vi "FTW-JSON-Core-GetFlattenedValue.vi"(0 "JSON Library Filepath":path, 5 "JSON Element":i64 format="%016x", 7 "LabVIEW Type":T1, 9 "Element Default Value":variant, 11 "error in":errorcluster, 12 "Encoding Flags":i64 format="%016x") -> (4 "Flattened Value":string, 15 "error out":errorcluster)   [LabVIEW 2014]
uses:
  reflection/FTW-Reflection-Types.ctl
  FTW-JSON-Core-Type.ctl
  error/FTW-ERR-ThrowError.vi
  lib/jansson/FTWLib-JSON-LibraryFilepath.vi
  error/FTW-ERR-NoErrorConstant.vi
  error/FTW-ERR-CallChain.vi
  string/FTW-STR-ReplaceWhitespace.vi
panel:
  # "Inputs"
  # "Outputs"
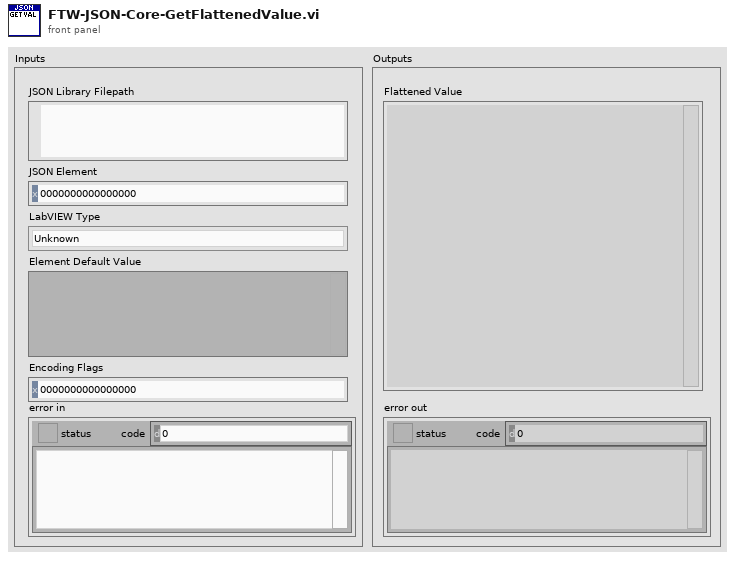
[diagram p1: front panel]
types:
  T1 = typedef "FTW-Reflection-Types.ctl" = enum16{"Unknown", "Void", "Array", "Cluster", "LVObject", "Boolean", "I8", "I16", "I32", "I64", "U8", "U16", "U32", "U64", "SGL", "DBL", "EXT", "CSG", "CDB", "CXT", "FXP", "EnumU8", "EnumU16", "EnumU32", "EnumU64", "SGLwithUnit", "DBLwithUnit", "EXTwithUnit", "CSGwithUnit", "CDBwithUnit", "CXTwithUnit", "String", "Path", "Picture", "Tag", "LVVariant", "Timestamp", "WaveformI8", "WaveformI16", "WaveformI32", "WaveformI64", "WaveformU8", "WaveformU16", "WaveformU32", "WaveformU64", "WaveformSGL", "WaveformDBL", "WaveformEXT", "WaveformCSG", "WaveformCDB", "WaveformCXT", "WaveformDigital", "WaveformUnknownType", "DigitalData", "DynamicData", "ExternalData", "FileByteStream", "TDMStream", "dotNET", "ActiveX", "VIServerReference", "VIReference", "ApplicationInstance", "Menu", "ConnectionDataSocket", "ConnectionVISA", "ConnectionBluetooth", "ConnectionIrDA", "ConnectionTCP", "ConnectionUDP", "ConnectionHTTPClient", "ConnectionFTP", "Occurrence", "Notifier", "Queue", "Rendezvous", "Semaphore", "RTFIFO", "EventPublisher", "EventRegistration", "EventCallback", "DataValueReference", "GenericClass", "GenericClassTag", "GenericClassDeepCopy", "GenericClassFlattened", "GenericClassTagFlattened", "GenericReferenceType", "WindowsRegistry", "OverloadedDatalogRef", "ReferenceUnknownType"}
  T2 = typedef "FTW-JSON-Core-Type.ctl" = enum16{"Object", "Array", "String", "Integer", "Floating Point", "true", "false", "null", "undefined"}
  T3 = cluster{"Element Name":string, "Element Type":T1, "Element Value":variant}[]
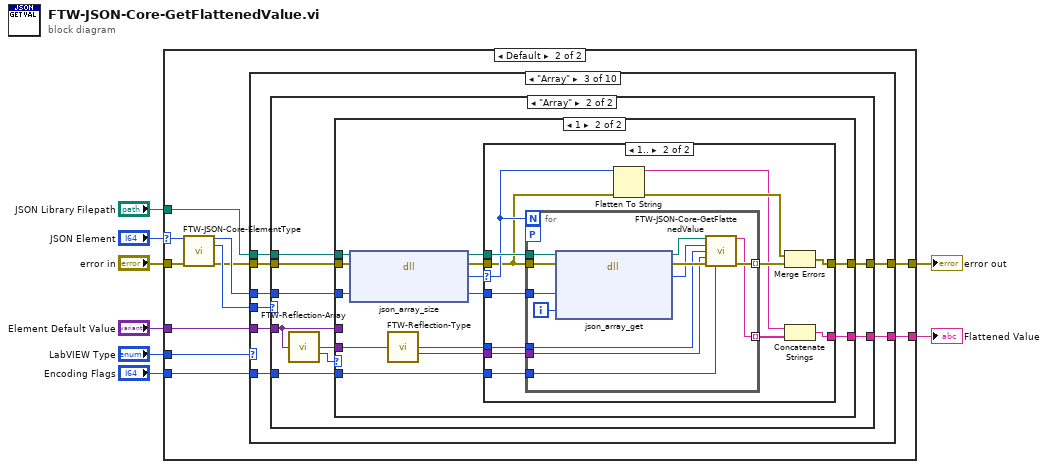
[diagram p0: block diagram]
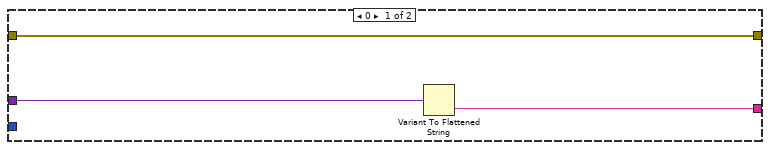
[diagram p2: hidden frame]
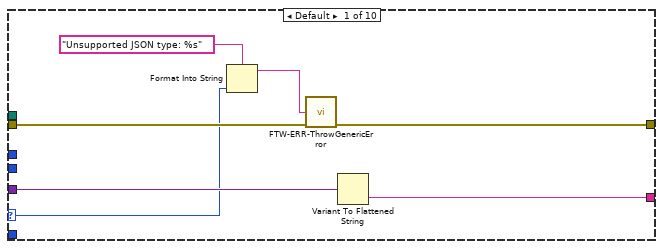
[diagram p3: hidden frame]
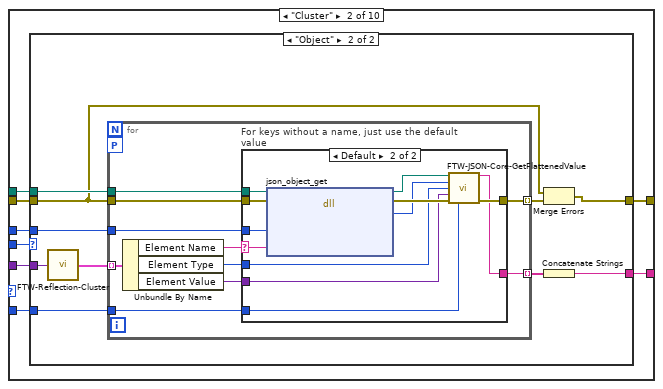
[diagram p4: hidden frame]
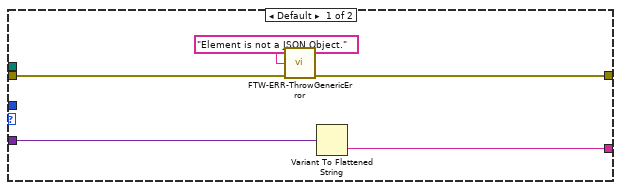
[diagram p5: hidden frame]
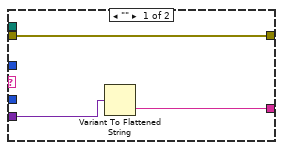
[diagram p6: hidden frame]
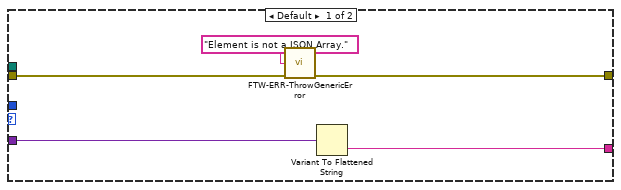
[diagram p7: hidden frame]
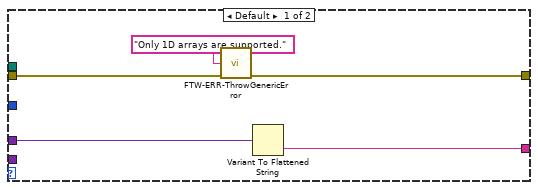
[diagram p8: hidden frame]
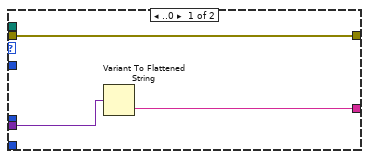
[diagram p9: hidden frame]
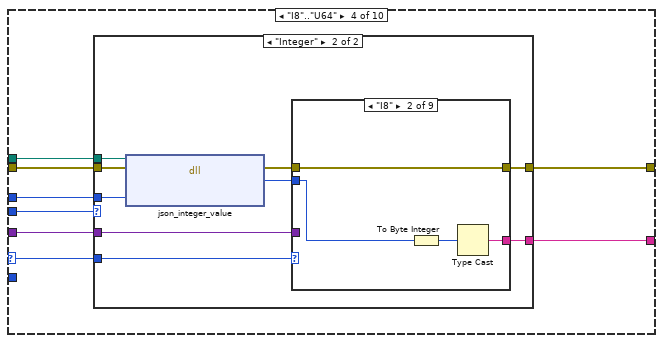
[diagram p10: hidden frame]
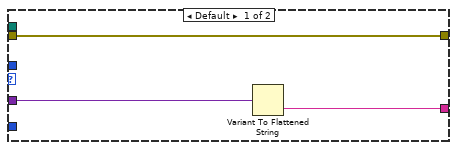
[diagram p11: hidden frame]
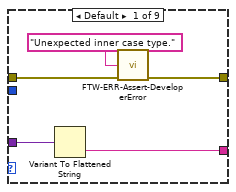
[diagram p12: hidden frame]
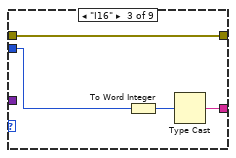
[diagram p13: hidden frame]
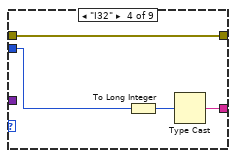
[diagram p14: hidden frame]
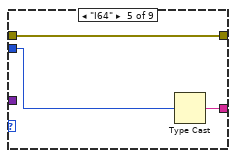
[diagram p15: hidden frame]
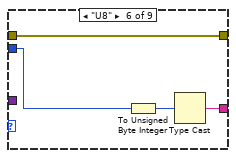
[diagram p16: hidden frame]
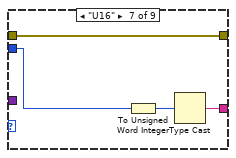
[diagram p17: hidden frame]
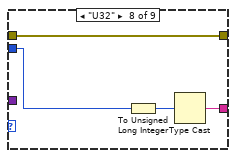
[diagram p18: hidden frame]
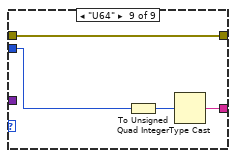
[diagram p19: hidden frame]
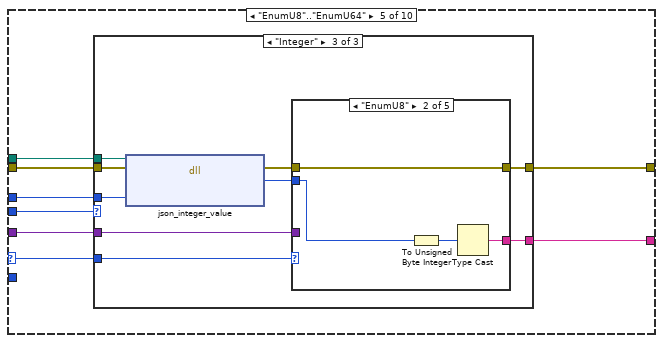
[diagram p20: hidden frame]
diagram:
  n1 = case shown="Default" "JSON Element" {
    selector: "JSON Element" -> [_ w15]
    tunnel: [w9 w22] -> w8
    tunnel: [w10 w21] -> w6
    tunnel: "LabVIEW Type" -> [_ w20]
    tunnel: "Element Default Value" -> [w11 w19]
    tunnel: "error in" -> [w9 w18]
    tunnel: "JSON Library Filepath" -> [_ w14]
    tunnel: "Encoding Flags" -> [_ w12]
    frame 0 {
      n2 = Variant To Flattened String(Variant=w11) -> (data string=w10:string)  [unwired: 1 out]
    }
    frame Default {
      n3 = call "FTW-JSON-Core-ElementType.vi"("JSON Element"=w15, "error in"=w18) -> ("JSON Element out"=w17:i64, "JSON Type"=w16:T2, "error out"=w13:errorcluster)  [unwired: 11 in]
      n4 = case shown="\"Array\"" w20 {
        selector: w20 -> [w23 _ _ w149 w205 w288 _ w364 _ _]
        tunnel: [w26 w33 w83 w146 w202 w285 w343 w361 w410 w441] -> w22
        tunnel: [w24 w36 w84 w151 w207 w290 w347 w366 w414 w444] -> w21
        tunnel: w13 -> [w27 w32 w82 w152 w208 w291 w348 w367 w415 w445]
        tunnel: w14 -> [_ w35 w80 w153 w209 w292 w349 w368 w416 _]
        tunnel: w17 -> [_ w34 w79 w148 w204 w287 w345 w363 w412 _]
        tunnel: w19 -> [w25 w37 w85 w150 w206 w289 w346 w365 w413 w443]
        tunnel: w16 -> [_ w31 w81 w147 w203 w286 w344 w362 w411 w442]
        tunnel: w12 -> [_ w30 w78 _ _ _ _ w360 _ _]
        frame Default {
          n5 = Format Into String(format string="Unsupported JSON type: %s", w23) -> (resulting string=w29:string)  [unwired: 2 in, 1 out]
          n6 = call "FTW-ERR-ThrowGenericError.vi"("Error Message"=w29, "error in"=w27) -> ("error out"=w26:errorcluster)  [unwired: 13 in]
          n7 = Variant To Flattened String(Variant=w25) -> (data string=w24:string)  [unwired: 1 out]
        }
        frame "Cluster" {
          n8 = case shown="\"Object\"" w31 {
            tunnel: w37 -> [w40 w51]
            tunnel: [w39 w49] -> w36
            tunnel: w35 -> [_ w48]
            tunnel: w34 -> [_ w46]
            tunnel: [w41 w45] -> w33
            tunnel: w32 -> [w42 w44]
            tunnel: w30 -> [_ w43]
            frame Default {
              n9 = call "FTW-ERR-ThrowGenericError.vi"("Error Message"="Element is not a JSON Object.", "error in"=w42) -> ("error out"=w41:errorcluster)  [unwired: 13 in]
              n10 = Variant To Flattened String(Variant=w40) -> (data string=w39:string)  [unwired: 1 out]
            }
            frame "Object" {
              n11 = call "FTW-Reflection-Cluster.vi"("Cluster"=w51) -> ("Cluster Elements"=w52:T3)  [unwired: 14 in]
              n12 = for {
                tunnel: w52 -> [w61] mode=indexing
                tunnel: [w58] -> w50 mode=indexing
                tunnel: w48 -> [w55]
                tunnel: w46 -> [w54]
                tunnel: w44 -> [w62]
                tunnel: [w56] -> w47 mode=indexing
                workers-P: _ -> [_]
                tunnel: w43 -> [w53]
                n13 = Unbundle By Name(w61) -> ("Element Name"=w60:string, "Element Type"=w57:T1, "Element Value"=w59:variant)
                n14 = case "For keys without a name, just use the default value" shown="Default" w60 {
                  selector: w60 -> [_ w73]
                  tunnel: w55 -> [_ w76]
                  tunnel: w62 -> [w63 w75]
                  tunnel: w59 -> [w65 w70]
                  tunnel: [w64 w71] -> w58
                  tunnel: w54 -> [_ w74]
                  tunnel: w57 -> [_ w69]
                  tunnel: [w63 w72] -> w56
                  tunnel: w53 -> [_ w66]
                  frame "" {
                    n15 = Variant To Flattened String(Variant=w65) -> (data string=w64:string)  [unwired: 1 out]
                  }
                  frame Default {
                    n16 = dll-call lib="?" fn="json_object_get"(path in=w76, error in=w75, "JSON Object Pointer"=w74, "Element Key"=w73) -> (path out=w67:path, error out=w77:errorcluster, "JSON Element Pointer"=w68:i64)  [unwired: 3 in]
                    n17 = call "FTW-JSON-Core-GetFlattenedValue.vi"("JSON Library Filepath"=w67, "JSON Element"=w68, "LabVIEW Type"=w69, "Element Default Value"=w70, "error in"=w77, "Encoding Flags"=w66) -> ("Flattened Value"=w71:string, "error out"=w72:errorcluster)  [unwired: 8 in]
                  }
                }
              }
              n18 = Merge Errors(w44, w47) -> (w45:errorcluster)
              n19 = Concatenate Strings(w50) -> (w49:string)
            }
          }
        }
        frame "Array" {
          n20 = case shown="\"Array\"" w81 {
            tunnel: w85 -> [w88 w92]
            tunnel: [w87 w99] -> w84
            tunnel: [w86 w98] -> w83
            tunnel: w82 -> [w89 w97]
            tunnel: w80 -> [_ w94]
            tunnel: w79 -> [_ w93]
            tunnel: w78 -> [_ w91]
            frame Default {
              n21 = call "FTW-ERR-ThrowGenericError.vi"("Error Message"="Element is not a JSON Array.", "error in"=w89) -> ("error out"=w86:errorcluster)  [unwired: 13 in]
              n22 = Variant To Flattened String(Variant=w88) -> (data string=w87:string)  [unwired: 1 out]
            }
            frame "Array" {
              n23 = call "FTW-Reflection-Array.vi"("Array"=w92) -> ("Default Array Element"=w96:variant, "Number of Dimensions"=w95:i32)  [unwired: 13 in]
              n24 = case shown="1" w95 {
                tunnel: [w101 w117] -> w99
                tunnel: [w102 w116] -> w98
                tunnel: w97 -> [w103 w115]
                tunnel: w96 -> [_ w109]
                tunnel: w94 -> [_ w114]
                tunnel: w93 -> [_ w113]
                tunnel: w92 -> [w100 _]
                tunnel: w91 -> [_ w105]
                frame Default {
                  n25 = call "FTW-ERR-ThrowGenericError.vi"("Error Message"="Only 1D arrays are supported.", "error in"=w103) -> ("error out"=w102:errorcluster)  [unwired: 13 in]
                  n26 = Variant To Flattened String(Variant=w100) -> (data string=w101:string)  [unwired: 1 out]
                }
                frame 1 {
                  n27 = dll-call lib="?" fn="json_array_size"(path in=w114, error in=w115, "Array Pointer"=w113) -> (path out=w112:path, error out=w110:errorcluster, "Array Size"=w106:i32, "Array Pointer"=w111:i64)  [unwired: 1 in]
                  n28 = call "FTW-Reflection-Type.vi"("Anything"=w109) -> ("LabVIEW Type"=w108:T1, "Variant Type and Value"=w107:variant)  [unwired: 12 in, 1 out]
                  n29 = case shown="1.." w106 {
                    selector: w106 -> [_ w125]
                    tunnel: [w120 w133] -> w117
                    tunnel: [w118 w132] -> w116
                    tunnel: w112 -> [_ w131]
                    tunnel: w111 -> [_ w130]
                    tunnel: w110 -> [w118 w122]
                    tunnel: w108 -> [_ w128]
                    tunnel: w107 -> [w119 w127]
                    tunnel: w105 -> [_ w121]
                    frame ..0 {
                      n30 = Variant To Flattened String(Variant=w119) -> (data string=w120:string)  [unwired: 1 out]
                    }
                    frame 1.. {
                      n31 = for {
                        N: w125 -> [_]
                        tunnel: w131 -> [w144]
                        tunnel: w130 -> [w142]
                        workers-P: _ -> [_]
                        tunnel: w122 -> [w143]
                        tunnel: [w140] -> w129 mode=indexing
                        tunnel: w128 -> [w137]
                        tunnel: w127 -> [w138]
                        tunnel: [w139] -> w126 mode=indexing
                        tunnel: w121 -> [w134]
                        i -> [w141]
                        n32 = dll-call lib="?" fn="json_array_get"(path in=w144, error in=w143, "Array Pointer"=w142, "Index"=w141) -> (path out=w135:path, error out=w145:errorcluster, "Array Element"=w136:i64)  [unwired: 3 in]
                        n33 = call "FTW-JSON-Core-GetFlattenedValue.vi"("JSON Library Filepath"=w135, "JSON Element"=w136, "LabVIEW Type"=w137, "Element Default Value"=w138, "error in"=w145, "Encoding Flags"=w134) -> ("Flattened Value"=w139:string, "error out"=w140:errorcluster)  [unwired: 8 in]
                      }
                      n34 = Flatten To String(anything=w125, error in (no error)=w122) -> (data string=w123:string, error out=w124:errorcluster)  [unwired: 2 in, 1 out]
                      n35 = Merge Errors(w124, w129) -> (w132:errorcluster)
                      n36 = Concatenate Strings(w123, w126) -> (w133:string)
                    }
                  }
                }
              }
            }
          }
        }
        frame "I8".."U64" {
          n37 = case shown="\"Integer\"" w147 {
            tunnel: w153 -> [_ w165]
            tunnel: w148 -> [_ w164]
            tunnel: w152 -> [w154 w163]
            tunnel: w150 -> [w156 w157]
            tunnel: [w155 w158] -> w151
            tunnel: [w154 w161] -> w146
            tunnel: w149 -> [_ w162]
            frame Default {
              n38 = Variant To Flattened String(Variant=w156) -> (data string=w155:string)  [unwired: 1 out]
            }
            frame "Integer" {
              n39 = dll-call lib="?" fn="json_integer_value"(path in=w165, error in=w163, "JSON Element Pointer"=w164) -> (error out=w160:errorcluster, "I64 Value"=w159:i64)  [unwired: 2 in, 1 out]
              n40 = case shown="\"I8\"" w162 {
                tunnel: [w169 w174 w178 w182 w185 w189 w193 w197 w201] -> w161
                tunnel: w160 -> [w170 w174 w178 w182 w185 w189 w193 w197 w201]
                tunnel: w159 -> [_ w172 w176 w180 w183 w187 w191 w195 w199]
                tunnel: [w166 w173 w177 w181 w184 w188 w192 w196 w200] -> w158
                tunnel: w157 -> [w167 _ _ _ _ _ _ _ _]
                frame Default {
                  n41 = Variant To Flattened String(Variant=w167) -> (data string=w166:string)  [unwired: 1 out]
                  n42 = call "FTW-ERR-Assert-DeveloperError.vi"("Reason this error should never happen"="Unexpected inner case type.", "error in"=w170) -> ("error out"=w169:errorcluster)  [unwired: 13 in]
                }
                frame "I8" {
                  n43 = To Byte Integer(number=w172) -> (8bit integer=w171:i8)
                  n44 = Type Cast(x=w171) -> (*(type *) &x=w173:string)  [unwired: 1 in]
                }
                frame "I16" {
                  n45 = To Word Integer(number=w176) -> (16bit integer=w175:i16)
                  n46 = Type Cast(x=w175) -> (*(type *) &x=w177:string)  [unwired: 1 in]
                }
                frame "I32" {
                  n47 = To Long Integer(number=w180) -> (32bit integer=w179:i32)
                  n48 = Type Cast(x=w179) -> (*(type *) &x=w181:string)  [unwired: 1 in]
                }
                frame "I64" {
                  n49 = Type Cast(x=w183) -> (*(type *) &x=w184:string)  [unwired: 1 in]
                }
                frame "U8" {
                  n50 = To Unsigned Byte Integer(number=w187) -> (unsigned 8bit integer=w186:u8)
                  n51 = Type Cast(x=w186) -> (*(type *) &x=w188:string)  [unwired: 1 in]
                }
                frame "U16" {
                  n52 = To Unsigned Word Integer(number=w191) -> (unsigned 16bit integer=w190:u16)
                  n53 = Type Cast(x=w190) -> (*(type *) &x=w192:string)  [unwired: 1 in]
                }
                frame "U32" {
                  n54 = To Unsigned Long Integer(number=w195) -> (unsigned 32bit integer=w194:u32)
                  n55 = Type Cast(x=w194) -> (*(type *) &x=w196:string)  [unwired: 1 in]
                }
                frame "U64" {
                  n56 = To Unsigned Quad Integer(1:w199) -> (0:w198:u64)
                  n57 = Type Cast(x=w198) -> (*(type *) &x=w200:string)  [unwired: 1 in]
                }
              }
            }
          }
        }
        frame "EnumU8".."EnumU64" {
          n58 = case shown="\"Integer\"" w203 {
            tunnel: w209 -> [_ w221 w261]
            tunnel: w204 -> [_ w220 w259]
            tunnel: w208 -> [w210 w219 w260]
            tunnel: w206 -> [w212 w213 w258]
            tunnel: [w211 w214 w255] -> w207
            tunnel: [w210 w217 w256] -> w202
            tunnel: w205 -> [_ w218 w257]
            frame Default {
              n59 = Variant To Flattened String(Variant=w212) -> (data string=w211:string)  [unwired: 1 out]
            }
            frame "String" {
              n60 = dll-call lib="?" fn="json_string_value"(path in=w221, error in=w219, "JSON Element Pointer"=w220) -> (error out=w216:errorcluster, "String Value"=w215:string)  [unwired: 2 in, 1 out]
              n61 = case shown="Default" w218 {
                tunnel: [w225 w233 w240 w247 w254] -> w217
                tunnel: w216 -> [w226 w233 w240 w247 w254]
                tunnel: w215 -> [_ w230 w237 w244 w251]
                tunnel: [w222 w229 w236 w243 w250] -> w214
                tunnel: w213 -> [w223 w232 w239 w246 w253]
                frame Default {
                  n62 = Variant To Flattened String(Variant=w223) -> (data string=w222:string)  [unwired: 1 out]
                  n63 = call "FTW-ERR-Assert-DeveloperError.vi"("Reason this error should never happen"="Unexpected inner case type.", "error in"=w226) -> ("error out"=w225:errorcluster)  [unwired: 13 in]
                }
                frame "EnumU8" {
                  n64 = call "FTW-Reflection-Enum.vi"("Enum"=w232) -> ("Enum Items"=w231:string[])  [unwired: 12 in, 2 out]
                  n65 = Search 1D Array(1D array=w231, element=w230) -> (index of element=w228:i32)  [unwired: 1 in]
                  n66 = To Unsigned Byte Integer(number=w228) -> (unsigned 8bit integer=w227:u8)
                  n67 = Type Cast(x=w227) -> (*(type *) &x=w229:string)  [unwired: 1 in]
                }
                frame "EnumU16" {
                  n68 = call "FTW-Reflection-Enum.vi"("Enum"=w239) -> ("Enum Items"=w238:string[])  [unwired: 12 in, 2 out]
                  n69 = Search 1D Array(1D array=w238, element=w237) -> (index of element=w235:i32)  [unwired: 1 in]
                  n70 = To Unsigned Word Integer(number=w235) -> (unsigned 16bit integer=w234:u16)
                  n71 = Type Cast(x=w234) -> (*(type *) &x=w236:string)  [unwired: 1 in]
                }
                frame "EnumU32" {
                  n72 = call "FTW-Reflection-Enum.vi"("Enum"=w246) -> ("Enum Items"=w245:string[])  [unwired: 12 in, 2 out]
                  n73 = Search 1D Array(1D array=w245, element=w244) -> (index of element=w242:i32)  [unwired: 1 in]
                  n74 = To Unsigned Long Integer(number=w242) -> (unsigned 32bit integer=w241:u32)
                  n75 = Type Cast(x=w241) -> (*(type *) &x=w243:string)  [unwired: 1 in]
                }
                frame "EnumU64" {
                  n76 = call "FTW-Reflection-Enum.vi"("Enum"=w253) -> ("Enum Items"=w252:string[])  [unwired: 12 in, 2 out]
                  n77 = Search 1D Array(1D array=w252, element=w251) -> (index of element=w249:i32)  [unwired: 1 in]
                  n78 = To Unsigned Quad Integer(1:w249) -> (0:w248:u64)
                  n79 = Type Cast(x=w248) -> (*(type *) &x=w250:string)  [unwired: 1 in]
                }
              }
            }
            frame "Integer" {
              n80 = dll-call lib="?" fn="json_integer_value"(path in=w261, error in=w260, "JSON Element Pointer"=w259) -> (error out=w263:errorcluster, "I64 Value"=w262:i64)  [unwired: 2 in, 1 out]
              n81 = case shown="\"EnumU8\"" w257 {
                tunnel: [w267 w272 w276 w280 w284] -> w256
                tunnel: w263 -> [w268 w272 w276 w280 w284]
                tunnel: w262 -> [_ w270 w274 w278 w282]
                tunnel: [w264 w271 w275 w279 w283] -> w255
                tunnel: w258 -> [w265 _ _ _ _]
                frame Default {
                  n82 = Variant To Flattened String(Variant=w265) -> (data string=w264:string)  [unwired: 1 out]
                  n83 = call "FTW-ERR-Assert-DeveloperError.vi"("Reason this error should never happen"="Unexpected inner case type.", "error in"=w268) -> ("error out"=w267:errorcluster)  [unwired: 13 in]
                }
                frame "EnumU8" {
                  n84 = To Unsigned Byte Integer(number=w270) -> (unsigned 8bit integer=w269:u8)
                  n85 = Type Cast(x=w269) -> (*(type *) &x=w271:string)  [unwired: 1 in]
                }
                frame "EnumU16" {
                  n86 = To Unsigned Word Integer(number=w274) -> (unsigned 16bit integer=w273:u16)
                  n87 = Type Cast(x=w273) -> (*(type *) &x=w275:string)  [unwired: 1 in]
                }
                frame "EnumU32" {
                  n88 = To Unsigned Long Integer(number=w278) -> (unsigned 32bit integer=w277:u32)
                  n89 = Type Cast(x=w277) -> (*(type *) &x=w279:string)  [unwired: 1 in]
                }
                frame "EnumU64" {
                  n90 = To Unsigned Quad Integer(1:w282) -> (0:w281:u64)
                  n91 = Type Cast(x=w281) -> (*(type *) &x=w283:string)  [unwired: 1 in]
                }
              }
            }
          }
        }
        frame "SGL".."EXT" {
          n92 = case shown="\"null\"" w286 {
            tunnel: w292 -> [_ w304 _]
            tunnel: w287 -> [_ w303 _]
            tunnel: w291 -> [w293 w302 w322]
            tunnel: w289 -> [w295 w296 w323]
            tunnel: [w294 w297 w324] -> w290
            tunnel: [w293 w300 w325] -> w285
            tunnel: w288 -> [_ w301 w326]
            frame Default {
              n93 = Variant To Flattened String(Variant=w295) -> (data string=w294:string)  [unwired: 1 out]
            }
            frame "Integer", "Floating Point" {
              n94 = dll-call lib="?" fn="json_number_value"(path in=w304, error in=w302, "JSON Element Pointer"=w303) -> (error out=w299:errorcluster, "DBL Value"=w298:dbl)  [unwired: 2 in, 1 out]
              n95 = case shown="\"SGL\"" w301 {
                tunnel: [w308 w313 w316 w320] -> w300
                tunnel: w299 -> [w309 w313 w316 w320]
                tunnel: w298 -> [_ w310 w314 w318]
                tunnel: [w305 w312 w315 w319] -> w297
                tunnel: w296 -> [w306 _ _ _]
                frame Default {
                  n96 = Variant To Flattened String(Variant=w306) -> (data string=w305:string)  [unwired: 1 out]
                  n97 = call "FTW-ERR-Assert-DeveloperError.vi"("Reason this error should never happen"="Unexpected inner case type.", "error in"=w309) -> ("error out"=w308:errorcluster)  [unwired: 13 in]
                }
                frame "SGL" {
                  n98 = To Single Precision Float(number=w310) -> (single precision float=w311:sgl)
                  n99 = Type Cast(x=w311) -> (*(type *) &x=w312:string)  [unwired: 1 in]
                }
                frame "DBL" {
                  n100 = Type Cast(x=w314) -> (*(type *) &x=w315:string)  [unwired: 1 in]
                }
                frame "EXT" {
                  n101 = To Extended Precision Float(1:w318) -> (0:w317:ext)
                  n102 = Type Cast(x=w317) -> (*(type *) &x=w319:string)  [unwired: 1 in]
                }
              }
            }
            frame "null" {
              n103 = case shown="\"SGL\"" w326 {
                tunnel: [w330 w335 w338 w342] -> w325
                tunnel: w322 -> [w331 w335 w338 w342]
                tunnel: nan ("DBL Value") -> [_ w332 w336 w340]
                tunnel: [w327 w334 w337 w341] -> w324
                tunnel: w323 -> [w328 _ _ _]
                frame Default {
                  n104 = Variant To Flattened String(Variant=w328) -> (data string=w327:string)  [unwired: 1 out]
                  n105 = call "FTW-ERR-Assert-DeveloperError.vi"("Reason this error should never happen"="Unexpected inner case type.", "error in"=w331) -> ("error out"=w330:errorcluster)  [unwired: 13 in]
                }
                frame "SGL" {
                  n106 = To Single Precision Float(number=w332) -> (single precision float=w333:sgl)
                  n107 = Type Cast(x=w333) -> (*(type *) &x=w334:string)  [unwired: 1 in]
                }
                frame "DBL" {
                  n108 = Type Cast(x=w336) -> (*(type *) &x=w337:string)  [unwired: 1 in]
                }
                frame "EXT" {
                  n109 = To Extended Precision Float(1:w340) -> (0:w339:ext)
                  n110 = Type Cast(x=w339) -> (*(type *) &x=w341:string)  [unwired: 1 in]
                }
              }
            }
          }
        }
        frame "Timestamp" {
          n111 = case shown="\"Floating Point\"" w344 {
            tunnel: w349 -> [_ w359]
            tunnel: w345 -> [_ w358]
            tunnel: w348 -> [w350 w357]
            tunnel: w346 -> [w352 _]
            tunnel: [w351 w355] -> w347
            tunnel: [w350 w356] -> w343
            frame Default {
              n112 = Variant To Flattened String(Variant=w352) -> (data string=w351:string)  [unwired: 1 out]
            }
            frame "Floating Point" {
              n113 = dll-call lib="?" fn="json_number_value"(path in=w359, error in=w357, "JSON Element Pointer"=w358) -> (error out=w356:errorcluster, "DBL Value"=w354:dbl)  [unwired: 2 in, 1 out]
              n114 = To Time Stamp(1:w354) -> (0:w353:timestamp)
              n115 = Type Cast(x=w353) -> (*(type *) &x=w355:string)  [unwired: 1 in]
            }
          }
        }
        frame "String".."Picture", "ConnectionVISA" {
          n116 = case shown="\"String\"" w362 {
            tunnel: w368 -> [_ _ w387]
            tunnel: w363 -> [w374 _ w386]
            tunnel: w367 -> [w375 w376 w385]
            tunnel: w365 -> [_ w378 w379]
            tunnel: [w371 w377 w380] -> w366
            tunnel: [w369 w376 w383] -> w361
            tunnel: w364 -> [_ _ w384]
            tunnel: w360 -> [w373 _ _]
            frame Default {
              n117 = call "FTW-JSON-Core-Serialize.vi"("JSON Object"=w374, "Encoding Flags"=w373, "error in"=w375) -> ("JSON String (UTF-8)"=w372:string, "error out"=w370:errorcluster)  [unwired: 10 in, 1 out]
              n118 = Flatten To String(anything=w372, error in (no error)=w370) -> (data string=w371:string, error out=w369:errorcluster)  [unwired: 2 in, 1 out]
            }
            frame "undefined" {
              n119 = Variant To Flattened String(Variant=w378) -> (data string=w377:string)  [unwired: 1 out]
            }
            frame "String" {
              n120 = dll-call lib="?" fn="json_string_value"(path in=w387, error in=w385, "JSON Element Pointer"=w386) -> (error out=w382:errorcluster, "String Value"=w381:string)  [unwired: 2 in, 1 out]
              n121 = case shown="\"Picture\"" w384 {
                tunnel: [w391 w395 w399 w404 w409] -> w383
                tunnel: w382 -> [w392 w396 w400 w405 w409]
                tunnel: w381 -> [_ w394 w398 w403 w408]
                tunnel: [w388 w393 w397 w402 w407] -> w380
                tunnel: w379 -> [w389 _ _ _ _]
                frame Default {
                  n122 = Variant To Flattened String(Variant=w389) -> (data string=w388:string)  [unwired: 1 out]
                  n123 = call "FTW-ERR-Assert-DeveloperError.vi"("Reason this error should never happen"="Unexpected inner case type.", "error in"=w392) -> ("error out"=w391:errorcluster)  [unwired: 13 in]
                }
                frame "String" {
                  n124 = Flatten To String(anything=w394, error in (no error)=w396) -> (data string=w393:string, error out=w395:errorcluster)  [unwired: 2 in, 1 out]
                }
                frame "ConnectionVISA" {
                  n125 = Flatten To String(anything=w398, error in (no error)=w400) -> (data string=w397:string, error out=w399:errorcluster)  [unwired: 2 in, 1 out]
                }
                frame "Path" {
                  n126 = String To Path(string=w403) -> (path=w401:path)
                  n127 = Flatten To String(anything=w401, error in (no error)=w405) -> (data string=w402:string, error out=w404:errorcluster)  [unwired: 2 in, 1 out]
                }
                frame "Picture" {
                  n128 = call "FTW-STR-Encode-Base64.vi"("Input"=w408, "Direction"=enum16{"Encode", "Decode"}."Decode") -> ("Output"=w407:string)
                }
              }
            }
          }
        }
        frame "FileByteStream".."ConnectionDataSocket", "ConnectionBluetooth".."ReferenceUnknownType" {
          n129 = case shown="\"String\"" w411 {
            tunnel: w416 -> [_ w431]
            tunnel: w412 -> [_ w430]
            tunnel: w415 -> [w417 w429]
            tunnel: w413 -> [w419 w424]
            tunnel: [w418 w426] -> w414
            tunnel: [w417 w422] -> w410
            frame Default {
              n130 = Variant To Flattened String(Variant=w419) -> (data string=w418:string)  [unwired: 1 out]
            }
            frame "String" {
              w427 = "0x%16x"  # Reference Format
              n131 = dll-call lib="?" fn="json_string_value"(path in=w431, error in=w429, "JSON Element Pointer"=w430) -> (error out=w421:errorcluster, "String Value"=w428:string, "JSON Element Pointer"=w420:i64)  [unwired: 1 in, 1 out]
              n132 = Scan From String(format string=w427, input string=w428, error in=w421, default 1=w420) -> (error out=w423:errorcluster, output 1=w425:i64)  [unwired: 1 in, 2 out]
              n133 = case shown="No Error" w423 {
                selector: w423 -> [w432 _]
                tunnel: [w436 w439] -> w426
                tunnel: w425 -> [w435 _]
                tunnel: w424 -> [_ w440]
                tunnel: [w432 w438] -> w422
                frame No Error {
                  n134 = Type Cast(type=refnum<k0> refnum, x=w435) -> (*(type *) &x=w434:refnum<k0>)
                  n135 = Type Cast(x=w434) -> (*(type *) &x=w436:string)  [unwired: 1 in]
                }
                frame Error {
                  n136 = Variant To Flattened String(Variant=w440) -> (data string=w439:string)  [unwired: 1 out]
                  n137 = call "FTW-ERR-ThrowGenericError.vi"("Error Message"="Unexpected reference format.") -> ("error out"=w438:errorcluster)  [unwired: 14 in]
                }
              }
            }
          }
        }
        frame "Boolean" {
          n138 = case shown="\"true\", \"false\"" w442 {
            selector: w442 -> [_ w451]
            tunnel: w445 -> [w446 w452]
            tunnel: w443 -> [w448 _]
            tunnel: [w447 w453] -> w444
            tunnel: [w446 w452] -> w441
            frame Default {
              n139 = Variant To Flattened String(Variant=w448) -> (data string=w447:string)  [unwired: 1 out]
            }
            frame "true", "false" {
              n140 = Equal?(x=w451, y=FTW-JSON-Core-Type."true" ("x")) -> (x = y?=w449:bool)
              n141 = Type Cast(x=w449) -> (*(type *) &x=w453:string)  [unwired: 1 in]
            }
          }
        }
      }
    }
  }
  "error out" <- w8
  "Flattened Value" <- w6
